vi "Take Image at Start and End.vi"() -> ()   [LabVIEW 2014]
uses:
  <vilib>/userdefined/High Color/IMAQdx.ctl
  Globals/Dynamic_call_global.ph.vi
  Globals/Meas_global.vi
panel:
  out "Time Interval (s)":dbl
  in  "VideoMode":u32=12
  in  "Interface name":T1="cam0"
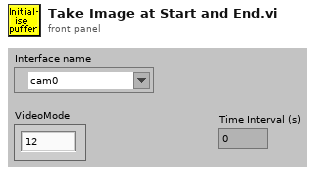
[diagram p1: front panel]
types:
  T1 = typedef "IMAQdx.ctl" = refnum<k21>
  T2 = typedef "Post_Process.ctl" = enum16{"Take New Data", "Post Process Raw Data File"}
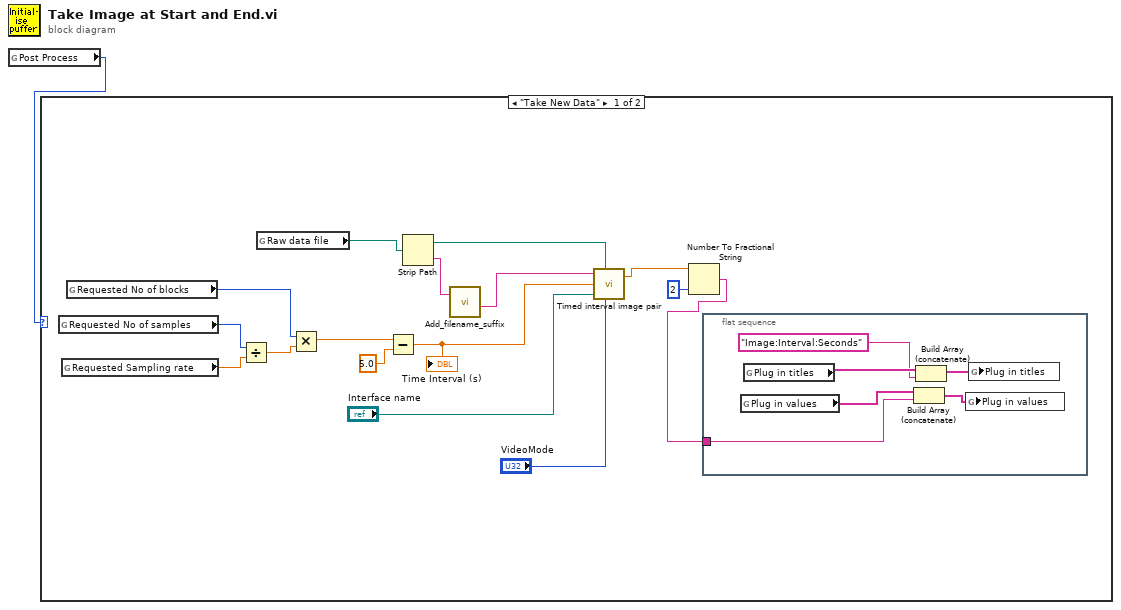
[diagram p0: block diagram]
diagram:
  n1 = global read "Meas_global.vi" "Post Process"() -> (w1:T2)
  n2 = case shown="\"Take New Data\"" w1 {
    frame "Take New Data" {
      n3 = global read "Meas_global.vi" "Requested No of samples"() -> (w13:i32)
      n4 = global read "Meas_global.vi" "Requested Sampling rate"() -> (w12:dbl)
      n5 = global read "Meas_global.vi" "Requested No of blocks"() -> (w10:i32)
      n6 = Divide(x=w13, y=w12) -> (x/y=w11:dbl)
      n7 = global read "Meas_global.vi" "Raw data file"() -> (w17:path)
      n8 = Multiply(x=w10, y=w11) -> (x*y=w5:dbl)
      n9 = Subtract(x=w5, y=5.0) -> (x-y=w3:dbl)
      "Time Interval (s)" <- w3
      n10 = Strip Path(path=w17) -> (stripped path=w16:path, name=w15:string)
      n11 = call "Add_filename_suffix.vi"("Filename"=w15) -> ("Base name"=w14:string)  [unwired: 1 in, 3 out]
      n12 = call "Timed interval image pair.vi"("Image name"=w14, "Image directory path"=w16, "Image pair interval (Sec)"=w3, "Interface name"="Interface name", "VideoMode"="VideoMode") -> ("Measured interval (s)"=w7:dbl)  [unwired: 1 out]
      n13 = Number To Fractional String(number=w7, precision (6)=i16 2) -> (F-format string=w2:string)  [unwired: 2 in]
      n14 = flat-sequence {
        tunnel: w2 -> [w18]
        frame #0 {
          n15 = global read "Dynamic_call_global.ph.vi" "Plug in values"() -> (w23:string[])
          n16 = global read "Dynamic_call_global.ph.vi" "Plug in titles"() -> (w22:string[])
          n17 = Build Array (concatenate)(w23, w18) -> (w21:string[])
          n18 = Build Array (concatenate)(w22, "Image:Interval:Seconds") -> (w20:string[])
          n19 = global write "Dynamic_call_global.ph.vi" "Plug in values"(w21) -> ()
          n20 = global write "Dynamic_call_global.ph.vi" "Plug in titles"(w20) -> ()
        }
      }
    }
    frame "Post Process Raw Data File", Default {
    }
  }
